vi "Create Gauss image.vi"() -> ()   [LabVIEW 2020, in "Camera Simulator.lvlib"]
uses:
  Camera Simulator.lvlib
panel:
  in  "Amplitude":i32=1000
  in  "1/e HWidth":dbl=10.0 format="%#_13g"
  in  "Image Y size":i32=1040
  in  "Center y":dbl=520.0 format="%#_13g"
  in  "Center x":dbl=520.0 format="%#_13g"
  in  "Image X size":i32=1040
  out "Image":T1(plugin-control)
  in  "File Path":path=path "C:/Users/user/Desktop/POLARIS Vision/Create SupeGauss/Suppergauss.png"
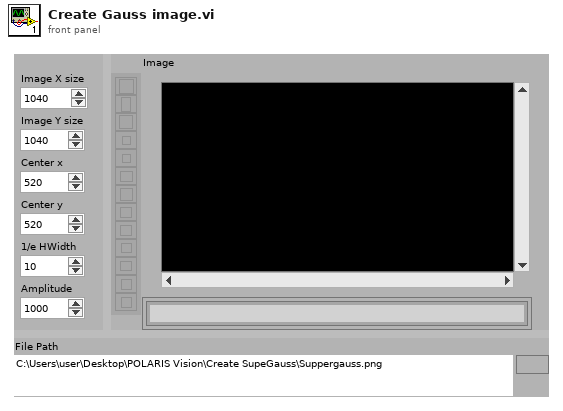
[diagram p1: front panel]
types:
  T1 = typedef "IMAQ Image.ctl" = refnum<image>
  T2 = typedef "Image Type" = u32
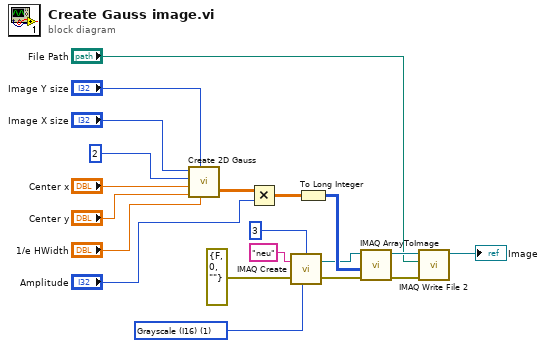
[diagram p0: block diagram]
diagram:
  w12 = T2 1 items=["Grayscale (U8)", "Grayscale (I16)", "Grayscale (SGL)", "Complex (CSG)", "RGB (U32)", "HSL (U32)", "RGB (U64)", "Grayscale (U16)"] ("Image Type")
  n1 = call "Create 2D Gauss.vi"("1/e HWidth"="1/e HWidth", "Y size"="Image Y size", "mitte y"="Center y", "mitte x"="Center x", "Order"=2, "X size"="Image X size") -> ("2D Gauss"=w10:sgl[][])  [unwired: 1 out]
  n2 = Multiply(x=w10, y="Amplitude") -> (x*y=w8:sgl[][])
  n3 = call "IMAQ Create"("Border Size"=3, "Image Name"="neu", "Image Type"=w12, "error in (no error)"=errorcluster {"status"=FALSE, "code"=0, "source"=""}) -> ("New Image"=w6:T1, "error out"=w4:errorcluster)  [unwired: 1 in]
  n4 = To Long Integer(number=w8) -> (32bit integer=w7:i32[][])
  n5 = call "IMAQ ArrayToImage"("error in (no error)"=w4, "Image Pixels (I16)"=w7, "Image"=w6) -> ("error out"=w3:errorcluster, "Image Out"=w5:T1)  [unwired: 7 in]
  n6 = call-poly "IMAQ Write File 2"("error in (no error)"=w3, "File Path"="File Path", "Image"=w5) -> ("Image Out (duplicate)"=→"Image":T1)  [unwired: 7 in, 1 out]
